vi "Instantiate_llm_openai_embed.vi"(0 "model_name":string(combo), 5 "openai_key":string, 11 "error in (no error)":errorcluster) -> (4 "llm_openai_embedding out":refnum<class "llm_gemini_embedding.lvclass">, 15 "error out":errorcluster)   [LabVIEW 2020, in "llm_gemini_embedding.lvclass"]
uses:
  llm_gemini_embedding.lvclass
  llm_gemini_embedding.lvclass/llm_gemini_embedding.ctl
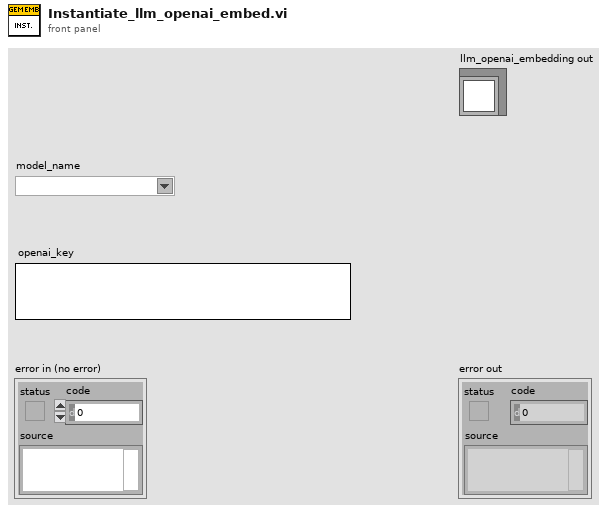
[diagram p1: front panel]
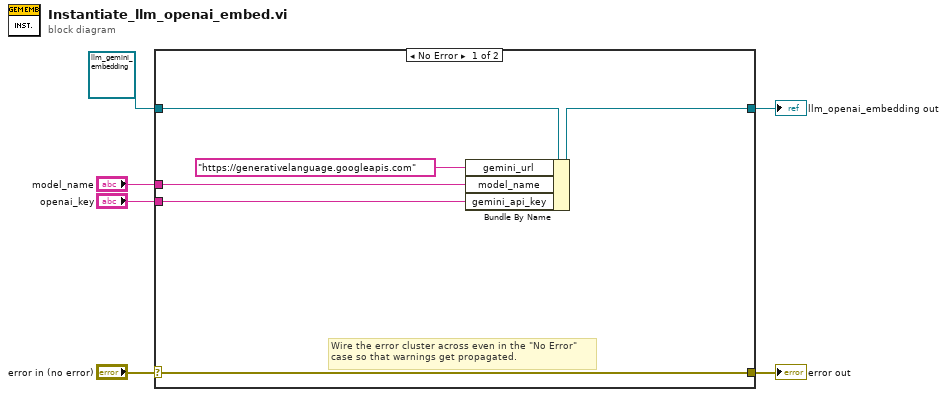
[diagram p0: block diagram]
diagram:
  n1 = case shown="No Error" "error in (no error)" {
    selector: "error in (no error)" -> [w12 w14]
    tunnel: [w12 w14] -> w5
    tunnel: [w7 w13] -> w3
    tunnel: refnum<class "llm_gemini_embedding.lvclass"> refnum ("llm_openai_embedding in") -> [w11 w13]
    tunnel: "openai_key" -> [w10 _]
    tunnel: "model_name" -> [w9 _]
    frame No Error {
      # "Wire the error cluster across even in the \"No Error\"\ncase so that warnings get propagated."
      n2 = Bundle By Name(cluster=w11, "gemini_url"="https://generativelanguage.googleapis.com" ("openai_url"), "model_name"=w9, "gemini_api_key"=w10) -> (w7:refnum<class "llm_gemini_embedding.lvclass">)
    }
    frame Error {
    }
  }
  "error out" <- w5
  "llm_openai_embedding out" <- w3
